vi "Translate Data.vi"(8 "error in (no error)":errorcluster, 10 "BufferIn":string, 11 "Alicat in":refnum<class "Alicat.lvclass">) -> (0 "error out":errorcluster, 2 "DataOut":refnum<class "Data.lvclass">, 3 "Alicat out":refnum<class "Alicat.lvclass">)   [LabVIEW 2015, in "Alicat.lvlib" / "Alicat.lvclass"]
doc: "VI used to translate the data buffer to something meaningful (implementation dependent). This VI must be overridden."
uses:
  Alicat.lvclass
  Reusable/Data/Data.lvclass
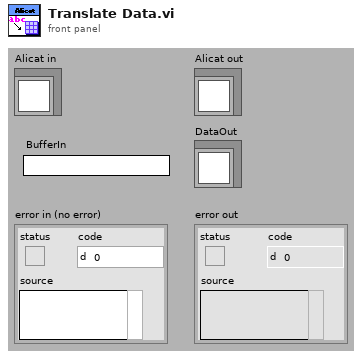
[diagram p1: front panel]
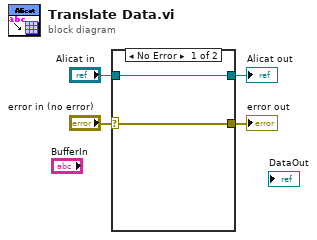
[diagram p0: block diagram]
diagram:
  n1 = case shown="No Error" "error in (no error)" {
    selector: "error in (no error)" -> [w5 w8]
    tunnel: [w5 w8] -> w3
    tunnel: [w6 w7] -> w1
    tunnel: "Alicat in" -> [w6 w7]
    frame No Error {
    }
    frame Error {
    }
  }
  "error out" <- w3
  "Alicat out" <- w1
